vi "mxwScript_API_XMLConnectToConPaneTerrminal.vi"(8 "error in (no error)":errorcluster, 9 "connection type":T1=enum."Recommended", 10 "connectorPaneTerminal":u32, 11 "connectorPaneName":string) -> (0 "error out":errorcluster, 3 "encoded connectorPaneName":string)   [LabVIEW 2020]
doc: "Create the encoded string to use for specifying the terminal location for connecting to the connector pane."
uses:
  codeGenAPISupport.llb/cgAPI_mxwScript_ConnPaneConnectionType.ctl
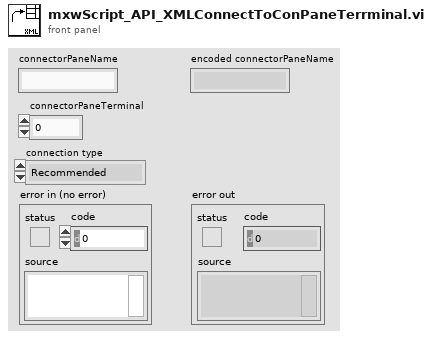
[diagram p1: front panel]
types:
  T1 = typedef "cgAPI_mxwScript_ConnPaneConnectionType.ctl" = enum16{"Invalid Wire Rule", "Required", "Recommended", "Optional", "Dynamic Dispatch"}
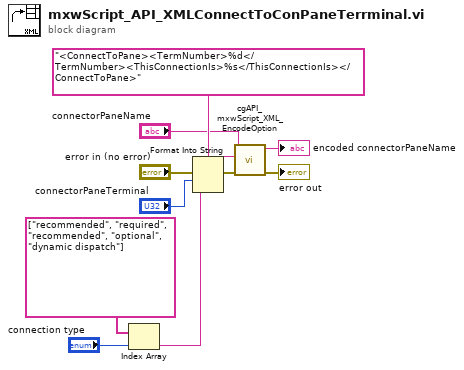
[diagram p0: block diagram]
diagram:
  n1 = Index Array(array=string[] ["recommended", "required", "recommended", "optional", "dynamic dispatch"], index="connection type") -> (element=w3:string)
  n2 = Format Into String(format string="<ConnectToPane><TermNumber>%d</TermNumber><ThisConnectionIs>%s</ThisConnectionIs></ConnectToPane>" ("control name"), error in="error in (no error)", "connectorPaneTerminal", w3) -> (resulting string=w6:string, error out=w8:errorcluster)  [unwired: 1 in]
  n3 = call "cgAPI_mxwScript_XML_EncodeOption.vi"("error in (no error)"=w8, "otherXML"=w6, "normalTextString"="connectorPaneName") -> ("error out"=→"error out":errorcluster, "encodedString"=→"encoded connectorPaneName":string)  [unwired: 7 out]
